vi "Create Plugin Configuration.vi"(6 "plugin timing":T2={"priority"=0, "decimation"=1, "offset"=0}, 9 "settings":T1, 10 "group configs":T5(array[cluster]), 11 "plugin class":string) -> (3 "Plugin Configuration":T6={"name"="", "class"="", "cycle timing"={"priority"=0, "decimation"=1, "offset"=0}, "Transfer Groups"=[], "settings"=[]})   [LabVIEW 2017]
uses:
  Builds/Data Sharing Framework/Windows/32/Data Sharing Framework Core/DSF Core.lvlibp/DSF Configuration API/Public/Controls/DSF Engine Plugin Configuration.ctl
  Builds/Data Sharing Framework/Windows/32/Data Sharing Framework Core/DSF Core.lvlibp/DSF Configuration API/Public/Controls/DSF Timing Info.ctl
  Builds/Data Sharing Framework/Windows/32/Data Sharing Framework Core/DSF Core.lvlibp/DSF Configuration API/Public/Controls/DSF Engine Transfer Group Configuration.ctl
  Builds/Data Sharing Framework/Windows/32/Data Sharing Framework Core/DSF Core.lvlibp/DSF Configuration API/Public/Controls/DSF Direction.ctl
  Builds/Data Sharing Framework/Windows/32/Data Sharing Framework Core/DSF Core.lvlibp/DSF Configuration API/Public/Controls/DSF Engine Transfer Configuration.ctl
  Builds/Data Sharing Framework/Windows/32/Data Sharing Framework Core/DSF Core.lvlibp/DSF Configuration API/Public/Controls/DSF Byte Order.ctl
  Builds/Data Sharing Framework/Windows/32/Data Sharing Framework Core/DSF Core.lvlibp/DSF Configuration API/Public/Controls/DSF Engine Channel Configuration.ctl
  Builds/Data Sharing Framework/Windows/32/Data Sharing Framework Core/DSF Core.lvlibp/DSF Configuration API/Public/Controls/DSF Data Type.ctl
  Builds/Data Sharing Framework/Windows/32/Data Sharing Framework Core/DSF Core.lvlibp/DSF Configuration API/Public/Controls/DSF Settings Info.ctl
  Builds/Data Sharing Framework/Windows/32/Data Sharing Framework Core/DSF Core.lvlibp
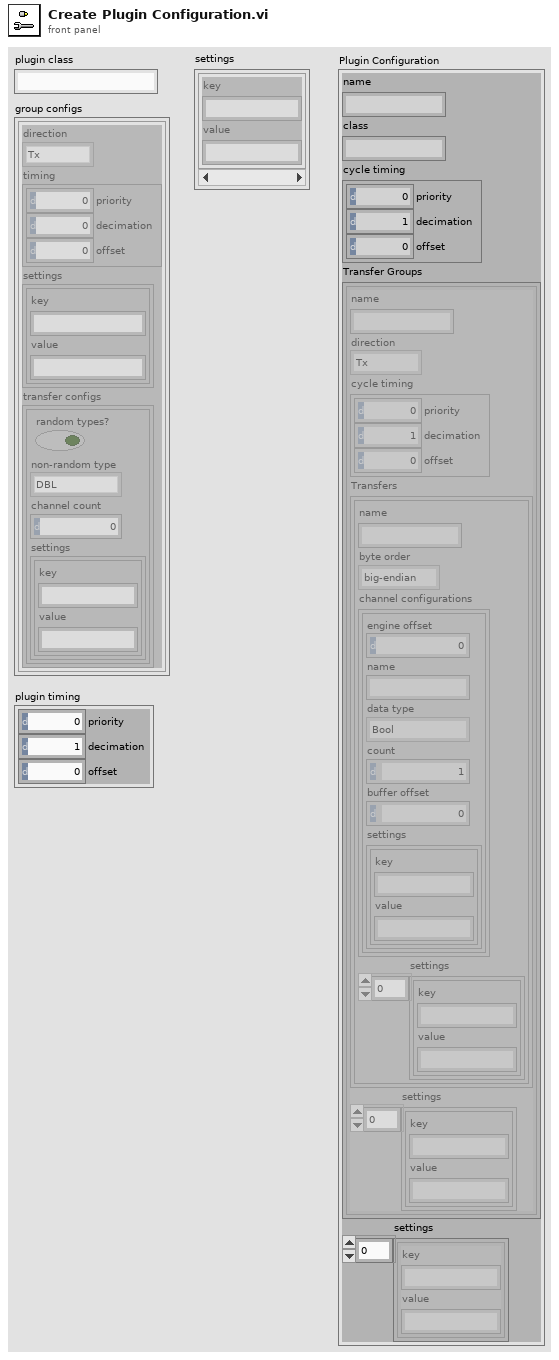
[diagram p1: front panel]
types:
  T1 = typedef "DSF Core.lvlibp/DSF Settings Info.ctl" = cluster{"key":string, "value":string}[]
  T2 = typedef "DSF Core.lvlibp/DSF Timing Info.ctl" = cluster{"priority":u64, "decimation":u64, "offset":u64}
  T3 = typedef "DSF Core.lvlibp/DSF Direction.ctl" = enum8{"Tx", "Rx"}
  T4 = typedef "DSF Core.lvlibp/DSF Data Type.ctl" = enum8{"Bool", "SGL", "DBL", "I8", "I16", "I32", "I64", "U8", "U16", "U32", "U64"}
  T5 = cluster{"direction":T3, "timing":T2, "settings":T1, "transfer configs":cluster{"random types?":bool, "non-random type":T4, "channel count":i32, "settings":T1}[]}[]
  T6 = typedef "DSF Core.lvlibp/DSF Engine Plugin Configuration.ctl" = cluster{"name":string, "class":string, "cycle timing":T2, "Transfer Groups":T7[], "settings":T1}
  T7 = typedef "DSF Core.lvlibp/DSF Engine Transfer Group Configuration.ctl" = cluster{"name":string, "direction":T3, "cycle timing":T2, "Transfers":T8[], "settings":T1}
  T8 = typedef "DSF Core.lvlibp/DSF Engine Transfer Configuration.ctl" = cluster{"name":string, "byte order":T9, "channel configurations":T10[], "settings":T1}
  T9 = typedef "DSF Core.lvlibp/DSF Byte Order.ctl" = enum8{"big-endian", "little-endian"}
  T10 = typedef "DSF Core.lvlibp/DSF Engine Channel Configuration.ctl" = cluster{"engine offset":u64, "name":string, "data type":T4, "count":u64, "buffer offset":u64, "settings":T1}
  T11 = cluster{"random types?":bool, "non-random type":T4, "channel count":i32, "settings":T1}[]
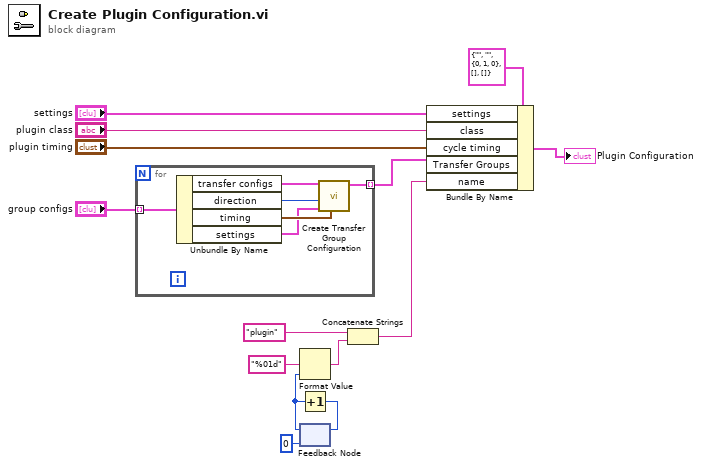
[diagram p0: block diagram]
diagram:
  n1 = for {
    tunnel: [w20] -> w3 mode=indexing
    tunnel: "group configs" -> [w19] mode=indexing
    n2 = Unbundle By Name(w19) -> ("transfer configs"=w15:T11, "direction"=w17:T3, "timing"=w18:T2, "settings"=w16:T1)
    n3 = call "Create Transfer Group Configuration.vi"("group timing (dec:1, off: 0)"=w18, "settings"=w16, "direction"=w17, "transfer configs"=w15) -> ("Transfer Group"=w20:T7)  [unwired: 7 in]
  }
  n4 = feedback #1(0) -> (w12:i32)
  n5 = Format Value(format string="%01d", value (0)=w12) -> (output string=w9:string)  [unwired: 1 in]
  n6 = Increment(x=w12) -> (x+1=w13:i32)
  n7 = feedback-in #1(w13) -> ()
  n8 = Concatenate Strings("plugin" ("name"), w9) -> (w6:string)
  n9 = Bundle By Name(cluster=T6 {"name"="", "class"="", "cycle timing"={"priority"=0, "decimation"=1, "offset"=0}, "Transfer Groups"=[], "settings"=[]} ("Plugins 2"), "settings"="settings", "class"="plugin class", "cycle timing"="plugin timing", "Transfer Groups"=w3, "name"=w6) -> (→"Plugin Configuration":T6)
